vi "Initialize Components UI.vi"(7 "user interface type":T2, 8 "error in (no error)":errorcluster, 11 "Item Ref in":T4 format="%.0x") -> (0 "error out":errorcluster, 1 "active vi":T3, 2 "User Interface Handler":refnum<class "User Interface Handler.lvclass">, 3 "Item Ref out":T4 format="%.0x", 4 "component settings":T1[](array[typedef]))   [LabVIEW 2019, in "DSF System Explorer.lvlib"]
uses:
  DSF System Explorer.lvlib
  Shared/DSF Shared.lvlib
  <vilib>/NI VeriStand/Custom Device API/Custom Device Item Ref.ctl
  <vilib>/NI VeriStand/Custom Device API/Custom Device API.lvlib
  DSF Core.lvlibp/Classes/User Interface Handler/User Interface Ref.ctl
  DSF Core.lvlibp/Classes/User Interface Handler/User Interface Handler.lvclass
  DSF Core.lvlibp/Classes/Component User Interface/UI Type.ctl
  DSF Core.lvlibp/Typedefs/DSF Settings Info.ctl
  DSF Core.lvlibp/Classes/User Interface/User Interface.lvclass
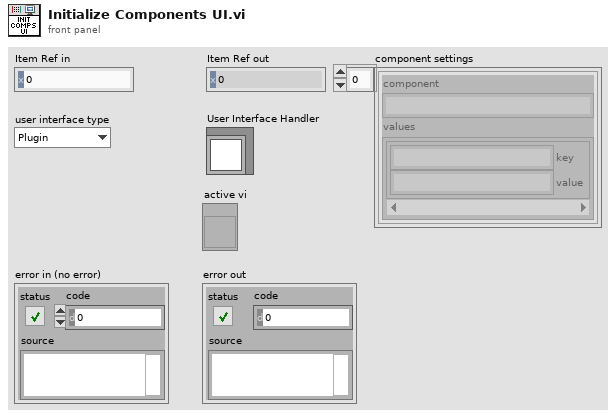
[diagram p1: front panel]
types:
  T1 = typedef "DSF Core.lvlibp/DSF Settings Info.ctl" = cluster{"component":string, "values":cluster{"key":string, "value":string}[]}
  T2 = typedef "DSF Core.lvlibp/Component User Interfaces.lvclass/UI Type.ctl" = enum16{"Plugin", "Thread", "Rx Group", "Tx Group", "Rx Transfer", "Tx Transfer", "Rx Channel", "Tx Channel"}
  T3 = typedef "DSF Core.lvlibp/User Interface Handler.lvclass/User Interface Ref.ctl" = refnum<vi>
  T4 = typedef "Custom Device API.lvlib/Custom Device Item Ref.ctl" = u64
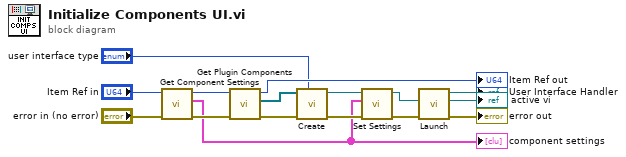
[diagram p0: block diagram]
diagram:
  n1 = call "Get Component Settings.vi"("error in (no error)"="error in (no error)", "Item Ref in"="Item Ref in") -> ("error out"=w15:errorcluster, "component settings"=w1:T1[], "Item Ref out"=w16:T4)  [unwired: 7 in]
  "component settings" <- w1
  n2 = call "Get Plugin Components.vi"("error in (no error)"=w15, "Item Ref in"=w16) -> ("error out"=w11:errorcluster, "Plugin Components"=w6:refnum<class "Component.lvclass">[], "Item Ref out"=→"Item Ref out":T4)  [unwired: 6 in, 1 out]
  n3 = call "Create.vi"("user interface type"="user interface type", "error in (no error)"=w11, "Components"=w6) -> ("error out"=w4:errorcluster, "Component Settings Editor"=w5:refnum<class "Component Settings Editor.lvclass">)  [unwired: 7 in]
  n4 = call "Set Settings.vi"("error in (no error)"=w4, "component settings"=w1, "Component Settings Editor in"=w5) -> ("error out"=w2:errorcluster, "Component Settings Editor out"=w3:refnum<class "Component Settings Editor.lvclass">)  [unwired: 7 in]
  n5 = call "Launch.vi"("error in (no error)"=w2, "User Interface"=w3) -> ("error out"=→"error out":errorcluster, "active vi"=→"active vi":T3, "User Interface Handler out"=→"User Interface Handler":refnum<class "User Interface Handler.lvclass">)  [unwired: 7 in]
